vi "GetParam.vi"(8 "error in (no error)":errorcluster caption="entrée d'erreur (pas d'erreur)", 11 "Regression.lvclass":refnum<class "Regression.lvclass">) -> (0 "error out":errorcluster caption="sortie d'erreur", 2 "make_regression":T1={"n_samples"=100, "n_features"=100, "n_informative"=10, "n_targets"=1, "bias"=0.0, "effective_rank"="None", "tail_strength"=0.5, "noise"=0.0, "shuffle"=TRUE, "random_state"=-1, "Returns"="X"} {"tail_strength" min=0.0 max=1.0; "n_targets" min=1; "n_features" min=1; "n_samples" min=1}, 3 "Regression.lvclass":refnum<class "Regression.lvclass">)   [LabVIEW 2020, in "Regression.lvclass"]
doc: "Get Parameters"
uses:
  Regression.lvclass
  Regression.lvclass/Regression.ctl
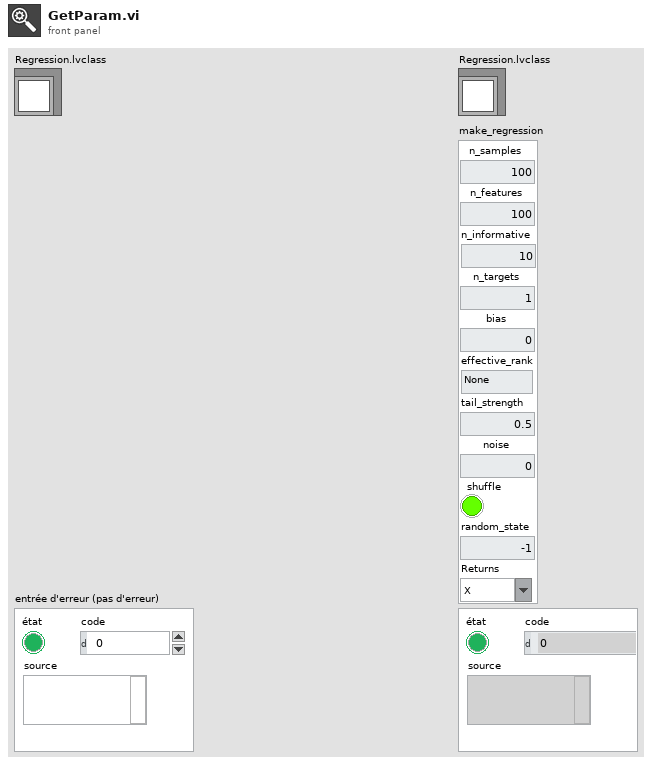
[diagram p1: front panel]
types:
  T1 = cluster{"n_samples":u32, "n_features":u32, "n_informative":u32, "n_targets":u32, "bias":dbl, "effective_rank":string, "tail_strength":dbl, "noise":dbl, "shuffle":bool, "random_state":i32, "Returns":string}
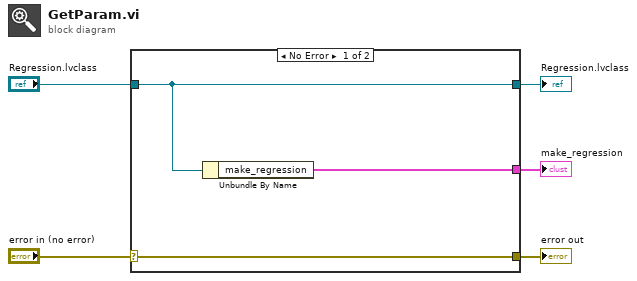
[diagram p0: block diagram]
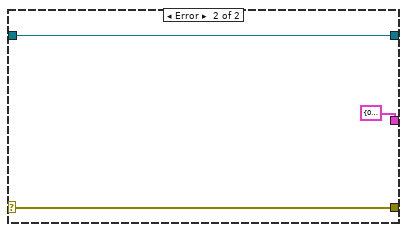
[diagram p2: hidden frame]
diagram:
  n1 = case shown="No Error" "error in (no error)" {
    selector: "error in (no error)" -> [w8 w10]
    tunnel: [w8 w10] -> w4
    tunnel: [w7 w11] -> w2
    tunnel: "Regression.lvclass" -> [w7 w11]
    tunnel: [w6 T1 {"n_samples"=0, "n_features"=0, "n_informative"=0, "n_targets"=0, "bias"=0.0, "effective_rank"="", "tail_strength"=0.0, "noise"=0.0, "shuffle"=FALSE, "random_state"=0, "Returns"=""} ("make_regression")] -> w1
    frame No Error {
      n2 = Unbundle By Name(w7) -> ("make_regression"=w6:T1)
    }
    frame Error {
    }
  }
  "error out" <- w4
  "Regression.lvclass" <- w2
  "make_regression" <- w1
